vi "shift spectra 3.vi"(0 "X name":string, 1 "2d intensity array":i32[][](array[numeric]), 2 "shift control":string(combo), 5 "Y name":string, 7 "Y range":i32[](array[numeric]), 9 "Y range Min":i32[](array[numeric]), 11 "Energy 2d gate in":T1, 12 "X range":i32[](array[numeric])) -> (3 "2d intensity array output":i32[][](array[numeric]), 4 "X name output":string, 6 "Y name  output":string, 8 "X range output":i32[](array[numeric]), 10 "Y range Max output":i32[](array[numeric]), 13 "Energy 2d gate out":T1, 15 "Y range Min output":i32[](array[numeric]))   [LabVIEW 2016]
doc: "Shift register for gate number 1"
uses:
  controls/energy 2d selection.ctl
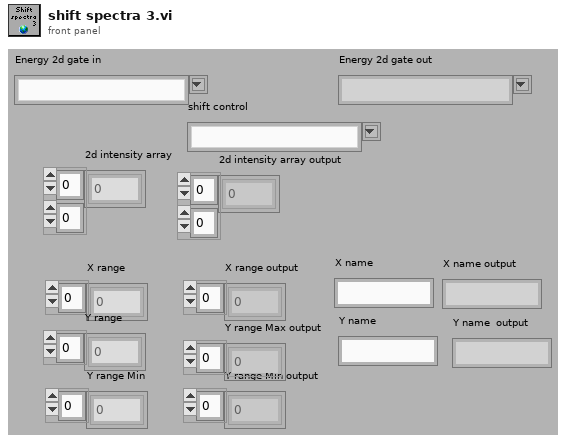
[diagram p1: front panel]
types:
  T1 = typedef "energy 2d selection.ctl" = string
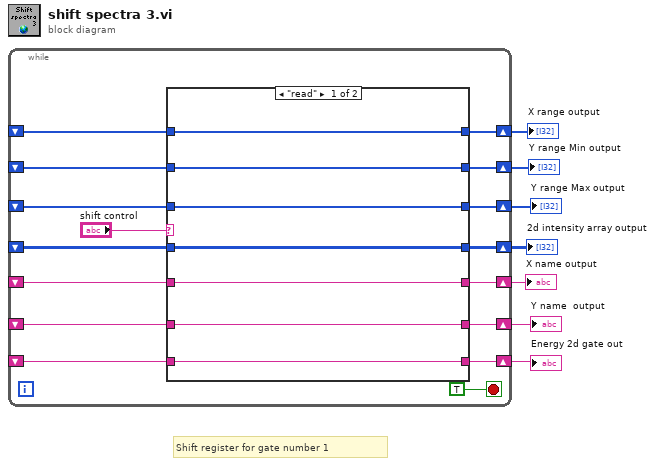
[diagram p0: block diagram]
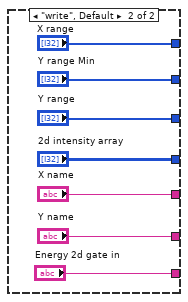
[diagram p2: hidden frame]
diagram:
  # "Shift register for gate number 1"
  n1 = while {
    shift-right: [w21] -> w7
    shift-left: _ -> [w15]
    shift-right: [w20] -> w6
    shift-left: _ -> [w14]
    shift-right: [w19] -> w5
    shift-left: _ -> [w13]
    shift-right: [w18] -> w4
    shift-left: _ -> [w12]
    shift-right: [w17] -> w3
    shift-left: _ -> [w11]
    shift-right: [w16] -> w2
    shift-left: _ -> [w10]
    shift-right: [w9] -> w1
    shift-left: _ -> [w8]
    stop <- TRUE ("stop") stop-if-true
    n2 = case shown="\"read\"" "shift control" {
      tunnel: [w30 "X range"] -> w21
      tunnel: [w29 "Y range Min"] -> w20
      tunnel: [w28 "Y range"] -> w19
      tunnel: [w27 "2d intensity array"] -> w18
      tunnel: [w26 "X name"] -> w17
      tunnel: [w25 "Y name"] -> w16
      tunnel: w15 -> [w30 _]
      tunnel: w14 -> [w29 _]
      tunnel: w13 -> [w28 _]
      tunnel: w12 -> [w27 _]
      tunnel: w11 -> [w26 _]
      tunnel: w10 -> [w25 _]
      tunnel: [w24 "Energy 2d gate in"] -> w9
      tunnel: w8 -> [w24 _]
      frame "read" {
      }
      frame "write", Default {
      }
    }
  }
  "X range output" <- w7
  "Y range Min output" <- w6
  "Y range Max output" <- w5
  "2d intensity array output" <- w4
  "X name output" <- w3
  "Y name  output" <- w2
  "Energy 2d gate out" <- w1
